vi "ItemByName.vi"(7 "LabVIEW Object Type":refnum<class>, 8 "error in (no error)":errorcluster, 10 "Name":string, 11 "CollectionByRef in":refnum<class "CollectionByRef.lvclass">) -> (0 "error out":errorcluster, 1 "found":bool, 2 "LabVIEW Object":refnum<class>, 3 "CollectionByRef out":refnum<class "CollectionByRef.lvclass">)   [LabVIEW 2021, in "Collection.lvlib" / "CollectionByRef.lvclass"]
uses:
  CollectionByRef.lvclass
  CollectionByRef.lvclass/CollectionByRef.ctl
  CollectionByValue/CollectionByValue.lvclass
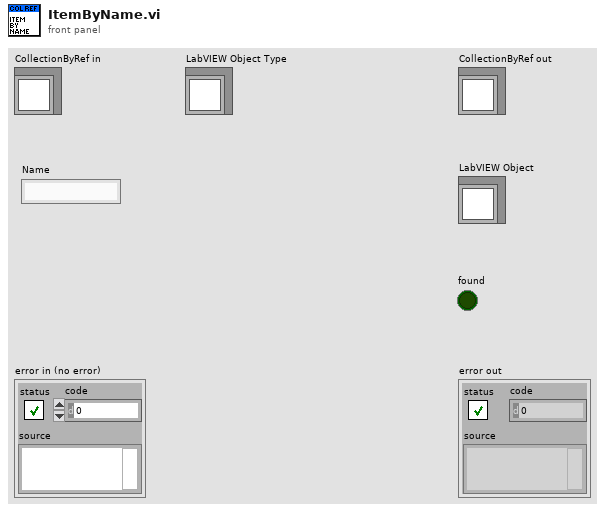
[diagram p1: front panel]
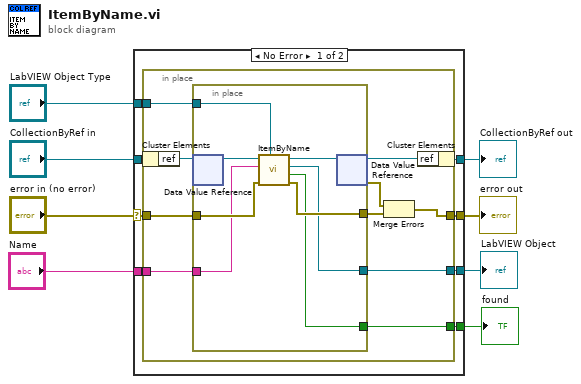
[diagram p0: block diagram]
diagram:
  n1 = case shown="No Error" "error in (no error)" {
    selector: "error in (no error)" -> [w14 w37]
    tunnel: [w13 w37] -> w5
    tunnel: [w15 w36] -> w7
    tunnel: "CollectionByRef in" -> [w16 w36]
    tunnel: "LabVIEW Object Type" -> [w12 w35]
    tunnel: "Name" -> [w11 _]
    tunnel: [w10 w35] -> w2
    tunnel: [w9 _] -> w1
    frame No Error {
      n2 = in-place {
        in-place-border: w14 -> [w24]
        in-place-border: [w21] -> w13
        in-place-border: w12 -> [w20]
        in-place-border: w11 -> [w19]
        in-place-border: [w18] -> w10
        in-place-border: [w17] -> w9
        n3 = in-place-cluster #1(w16) -> ("ref"=w25:refnum<data-value>)
        n4 = in-place {
          in-place-border: w24 -> [w32]
          in-place-border: [w31] -> w22
          in-place-border: w20 -> [w30]
          in-place-border: w19 -> [w29]
          in-place-border: [w28] -> w18
          in-place-border: [w27] -> w17
          n5 = in-place-dvr #2(w25) -> (w34:refnum<class "CollectionByValue.lvclass">)  [unwired: 1 out]
          n6 = call "ItemByName.vi"("LabVIEW Object Type"=w30, "error in (no error)"=w32, "Name"=w29, "Collection in"=w34) -> ("error out"=w31:errorcluster, "found?"=w27:bool, "LabVIEW Object"=w28:refnum<class>, "Collection out"=w33:refnum<class "CollectionByValue.lvclass">)  [unwired: 4 in]
          n7 = in-place-dvr #2(w33) -> (w26:refnum<data-value>, w23:errorcluster)
        }
        n8 = Merge Errors(w23, w22) -> (w21:errorcluster)
        n9 = in-place-cluster #1("ref"=w26) -> (w15:refnum<class "CollectionByRef.lvclass">)
      }
    }
    frame Error {
    }
  }
  "error out" <- w5
  "CollectionByRef out" <- w7
  "LabVIEW Object" <- w2
  "found" <- w1
